vi "CRYCurve Library Global.vi"() -> ()   [LabVIEW 2013]
uses:
  CRYSystem/Typedef Control/CRYImageData.ctl
  Control/CRYCurveLib Info Cluster.ctl
panel:
  in  "RedoProtectedData":T1
  in  "RedoFlag":bool
  in  "Work Data path":path
  out "ReplaceNames":T2
  in  "WavesOrder":i32[](array[numeric])
  in  "ResultsOrder":i32[](array[numeric])
  in  "ValuesOrder":i32[](array[numeric])
  in  "CruvesOrder":i32[](array[numeric])
  in  "StepOK":bool
  in  "StepClosebyOKCancel":bool
  in  "DiffLangSequenceLoad":bool
  in  "ProtectDataStepName":string
  out "ProtectDataStepNo":i32
  in  "CurveLib Info":T3
  in  "OverwriteStatus":string
  in  "OverwriteStart":bool
  out "OverwriteNumber":i32
  out "LoopIndexTreeIndex":i32
  out "ProtectTreeIndex":i32
  in  "WFM Items":T4(array[cluster])
  in  "Result Items":T4(array[cluster])
  in  "Value Items":T4(array[cluster])
  in  "Curve Items":T4(array[cluster])
  out "Probe Number":i32
  in  "Drag into CurLib":cluster{"DataName":string, "DragData":variant}
  in  "Curves Tree":refnum<vi>
  in  "Values Tree":refnum<vi>
  in  "Results Tree":refnum<vi>
  in  "CurLib Type":string
  in  "Curve Library VI":refnum<vi>
  out "Warkmark Image":T5[](array[typedef])=[{"image type"=0, "image depth"=32, "image"=array[2604 elements], "mask"=[255, 255, 255, 254, 255, 255, 255, 254, 255, 255, 255, 254, 255, 255, 255, 254, 255, 255, 255, 254, 255, 255, 255, 254, 255, 255, 255, 254, 255, 255, 255, 254, 255, 255, 255, 254, 255, 255, 255, 254, 255, 255, 255, 254, 255, 255, 255, 254, 255, 255, 255, 254, 255, 255, 255, 254, 255, 255, 255, 254, 255, 255, 255, 254, 255, 255, 255, 254, 255, 255, 255, 254, 255, 255, 255, 254, 255, 255, 255, 254, 255, 255, 255, 254], "colors"=[], "Rectangle"={"left"=0, "top"=0, "right"=31, "bottom"=21}}, {"image type"=0, "image depth"=32, "image"=array[3700 elements], "mask"=[255, 255, 255, 255, 248, 0, 255, 255, 255, 255, 248, 0, 255, 255, 255, 255, 248, 0, 255, 255, 255, 255, 248, 0, 255, 255, 255, 255, 248, 0, 255, 255, 255, 255, 248, 0, 255, 255, 255, 255, 248, 0, 255, 255, 255, 255, 248, 0, 255, 255, 255, 255, 248, 0, 255, 255, 255, 255, 248, 0, 255, 255, 255, 255, 248, 0, 255, 255, 255, 255, 248, 0, 255, 255, 255, 255, 248, 0, 255, 255, 255, 255, 248, 0, 255, 255, 255, 255, 248, 0, 255, 255, 255, 255, 248, 0, 255, 255, 255, 255, 248, 0, 255, 255, 255, 255, 248, 0, 255, 255, 255, 255, 248, 0, 255, 255, 255, 255, 248, 0, 255, 255, 255, 255, 248, 0, 255, 255, 255, 255, 248, 0, 255, 255, 255, 255, 248, 0, 255, 255, 255, 255, 248, 0, 255, 255, 255, 255, 248, 0], "colors"=[], "Rectangle"={"left"=0, "top"=0, "right"=37, "bottom"=25}}, {"image type"=0, "image depth"=32, "image"=array[5704 elements], "mask"=[255, 255, 255, 255, 255, 252, 255, 255, 255, 255, 255, 252, 255, 255, 255, 255, 255, 252, 255, 255, 255, 255, 255, 252, 255, 255, 255, 255, 255, 252, 255, 255, 255, 255, 255, 252, 255, 255, 255, 255, 255, 252, 255, 255, 255, 255, 255, 252, 255, 255, 255, 255, 255, 252, 255, 255, 255, 255, 255, 252, 255, 255, 255, 255, 255, 252, 255, 255, 255, 255, 255, 252, 255, 255, 255, 255, 255, 252, 255, 255, 255, 255, 255, 252, 255, 255, 255, 255, 255, 252, 255, 255, 255, 255, 255, 252, 255, 255, 255, 255, 255, 252, 255, 255, 255, 255, 255, 252, 255, 255, 255, 255, 255, 252, 255, 255, 255, 255, 255, 252, 255, 255, 255, 255, 255, 252, 255, 255, 255, 255, 255, 252, 255, 255, 255, 255, 255, 252, 255, 255, 255, 255, 255, 252, 255, 255, 255, 255, 255, 252, 255, 255, 255, 255, 255, 252, 255, 255, 255, 255, 255, 252, 255, 255, 255, 255, 255, 252, 255, 255, 255, 255, 255, 252, 255, 255, 255, 255, 255, 252, 255, 255, 255, 255, 255, 252], "colors"=[], "Rectangle"={"left"=0, "top"=0, "right"=46, "bottom"=31}}, {"image type"=0, "image depth"=32, "image"=array[2604 elements], "mask"=[255, 255, 255, 254, 255, 255, 255, 254, 255, 255, 253, 254, 251, 255, 255, 190, 255, 255, 255, 238, 255, 255, 255, 246, 255, 255, 255, 254, 255, 255, 255, 254, 255, 255, 255, 254, 255, 255, 255, 254, 255, 255, 255, 254, 255, 255, 255, 254, 255, 255, 255, 254, 255, 255, 255, 254, 255, 255, 255, 250, 255, 255, 255, 246, 247, 255, 255, 222, 253, 255, 255, 254, 255, 255, 255, 254, 255, 255, 255, 254, 255, 255, 255, 254], "colors"=[], "Rectangle"={"left"=0, "top"=0, "right"=31, "bottom"=21}}, {"image type"=0, "image depth"=32, "image"=array[3700 elements], "mask"=[255, 255, 255, 255, 248, 0, 255, 255, 143, 255, 248, 0, 255, 207, 255, 159, 248, 0, 254, 127, 255, 243, 248, 0, 249, 255, 255, 252, 248, 0, 247, 255, 255, 255, 120, 0, 239, 255, 255, 255, 152, 0, 255, 255, 255, 255, 216, 0, 255, 255, 255, 255, 248, 0, 255, 255, 255, 255, 248, 0, 255, 255, 255, 255, 248, 0, 255, 255, 255, 255, 248, 0, 255, 255, 255, 255, 248, 0, 255, 255, 255, 255, 248, 0, 255, 255, 255, 255, 248, 0, 255, 255, 255, 255, 248, 0, 191, 255, 255, 255, 232, 0, 223, 255, 255, 255, 216, 0, 239, 255, 255, 255, 184, 0, 247, 255, 255, 255, 120, 0, 253, 255, 255, 253, 248, 0, 255, 63, 255, 231, 248, 0, 255, 227, 254, 127, 248, 0, 255, 255, 255, 255, 248, 0, 255, 255, 255, 255, 248, 0], "colors"=[], "Rectangle"={"left"=0, "top"=0, "right"=37, "bottom"=25}}, {"image type"=0, "image depth"=32, "image"=array[5704 elements], "mask"=[255, 255, 255, 255, 255, 252, 255, 255, 255, 255, 255, 252, 255, 252, 31, 224, 255, 252, 255, 227, 255, 255, 31, 252, 255, 63, 255, 255, 227, 252, 252, 255, 255, 255, 252, 252, 251, 255, 255, 255, 255, 124, 247, 255, 255, 255, 255, 156, 239, 255, 255, 255, 255, 204, 255, 255, 255, 255, 255, 236, 255, 255, 255, 255, 255, 252, 255, 255, 255, 255, 255, 252, 255, 255, 255, 255, 255, 252, 255, 255, 255, 255, 255, 252, 255, 255, 255, 255, 255, 252, 255, 255, 255, 255, 255, 252, 255, 255, 255, 255, 255, 252, 255, 255, 255, 255, 255, 252, 255, 255, 255, 255, 255, 252, 255, 255, 255, 255, 255, 252, 191, 255, 255, 255, 255, 244, 223, 255, 255, 255, 255, 236, 239, 255, 255, 255, 255, 220, 247, 255, 255, 255, 255, 60, 249, 255, 255, 255, 254, 124, 254, 127, 255, 255, 249, 252, 255, 159, 255, 255, 199, 252, 255, 241, 255, 254, 63, 252, 255, 255, 0, 3, 255, 252, 255, 255, 255, 255, 255, 252, 255, 255, 255, 239, 255, 252], "colors"=[], "Rectangle"={"left"=0, "top"=0, "right"=46, "bottom"=31}}]
  out "XYGraphNumber":u32
  out "Frequency Color":u32[](array[numeric])
  out "WaveGraphNumber":u32
  in  "Graph Inner Click":bool
  out "AutoProtected Index":T6
  in  "UndoAutoProtect Button":refnum<vi>
  in  "AutoProtect Button":refnum<vi>
  out "Curve Image Data":T5[](array[typedef])
  in  "Type":enum16{"Curves", "Values", "Results", "WFM"}(ring)
  out "Wave Count":i32
  out "Curve Count":i32
  out "Color Palette":u32[](array[numeric])
  in  "Curve Library Global Inserting":bool
  in  "Curve Library Loading":bool
  in  "Curve Library Exist":bool
  out "Probe Array":T7(array[cluster])
  in  "Protect Button":refnum<vi>
  in  "Delete Button":refnum<vi>
  in  "Save Button":refnum<vi>
  in  "Open Button":refnum<vi>
  in  "Curve Library Tab":refnum<vi>
  in  "WFM Tree":refnum<vi>
  # "MultiListBox Control Reference"
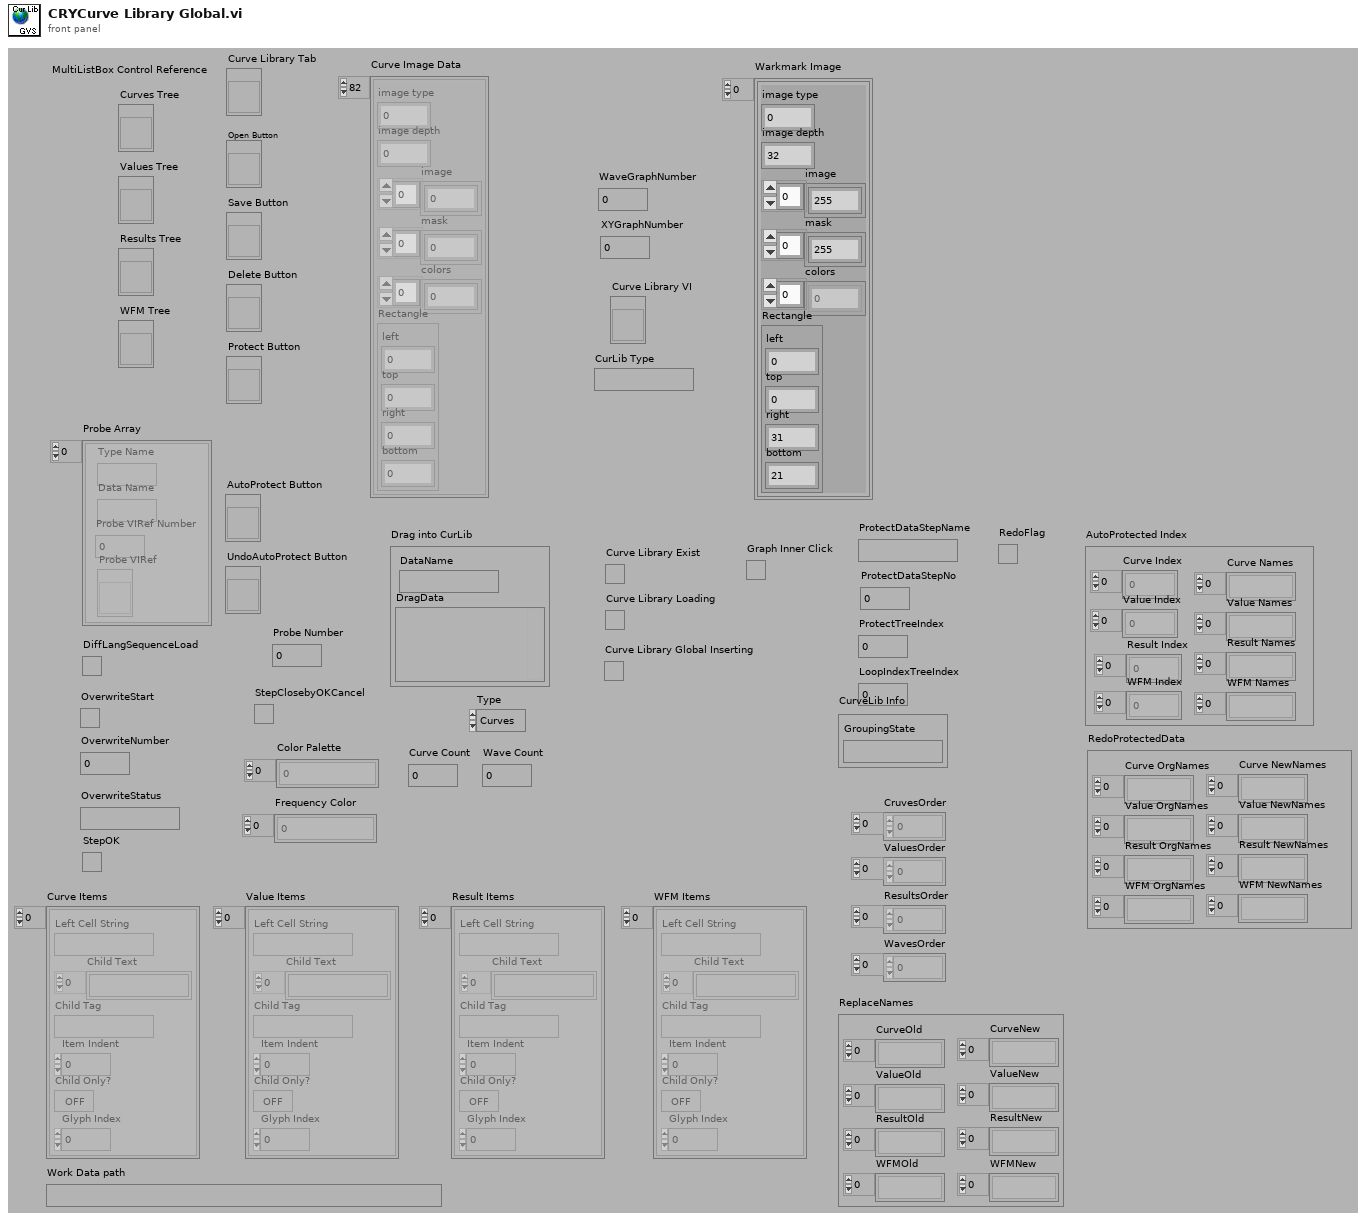
[diagram p1: front panel]
types:
  T1 = cluster{"Curve OrgNames":string[], "Value OrgNames":string[], "Result OrgNames":string[], "WFM OrgNames":string[], "Curve NewNames":string[], "Value NewNames":string[], "Result NewNames":string[], "WFM NewNames":string[]}
  T2 = cluster{"CurveOld":string[], "ValueOld":string[], "ResultOld":string[], "WFMOld":string[], "CurveNew":string[], "ValueNew":string[], "ResultNew":string[], "WFMNew":string[]}
  T3 = typedef "CRYCurveLib Info Cluster.ctl" = cluster{"GroupingState":string}
  T4 = cluster{"Left Cell String":string, "Child Text":string[], "Child Tag":string, "Item Indent":i32, "Child Only?":bool, "Glyph Index":i32}[]
  T5 = typedef "CRYImageData.ctl" = cluster{"image type":i32, "image depth":i32, "image":u8[], "mask":u8[], "colors":u32[], "Rectangle":cluster{"left":i16, "top":i16, "right":i16, "bottom":i16}}
  T6 = cluster{"Curve Index":i32[], "Value Index":i32[], "Result Index":i32[], "WFM Index":i32[], "Curve Names":string[], "Value Names":string[], "Result Names":string[], "WFM Names":string[]}
  T7 = cluster{"Type Name":string, "Data Name":string, "Probe VIRef Number":i32, "Probe VIRef":refnum<vi>}[]
diagram:
